vi "WheelShooter Load Data.vi"(1 "error in":errorcluster, 2 "Range":dbl) -> (0 "cluster":T9)   [LabVIEW 2015]
uses:
  <vilib>/Rock Robotics/WPI/MotorControl/WPI_MotorControlDeviceRef.ctl
  <vilib>/Rock Robotics/WPI/MotorControl/WPI_MotorControlType.ctl
  <vilib>/Rock Robotics/SystemInterfaces/DIO/FPGA_DIOPWMChannel.ctl
  <vilib>/Rock Robotics/WPI/PWM/WPI_PWMDeadband.ctl
  <vilib>/Rock Robotics/WPI/CAN/Jaguar/SubVIs/WPI_CANJaguar_ControlMode.ctl
  <vilib>/Rock Robotics/WPI/CAN/TalonSRX/WPI_CANTalonSRX_APIControlMode.ctl
  <vilib>/Rock Robotics/WPI/PWM/Servo/WPI_ServoDeviceRef.ctl
  <vilib>/Utility/file.llb/Read Delimited Spreadsheet (DBL).vi
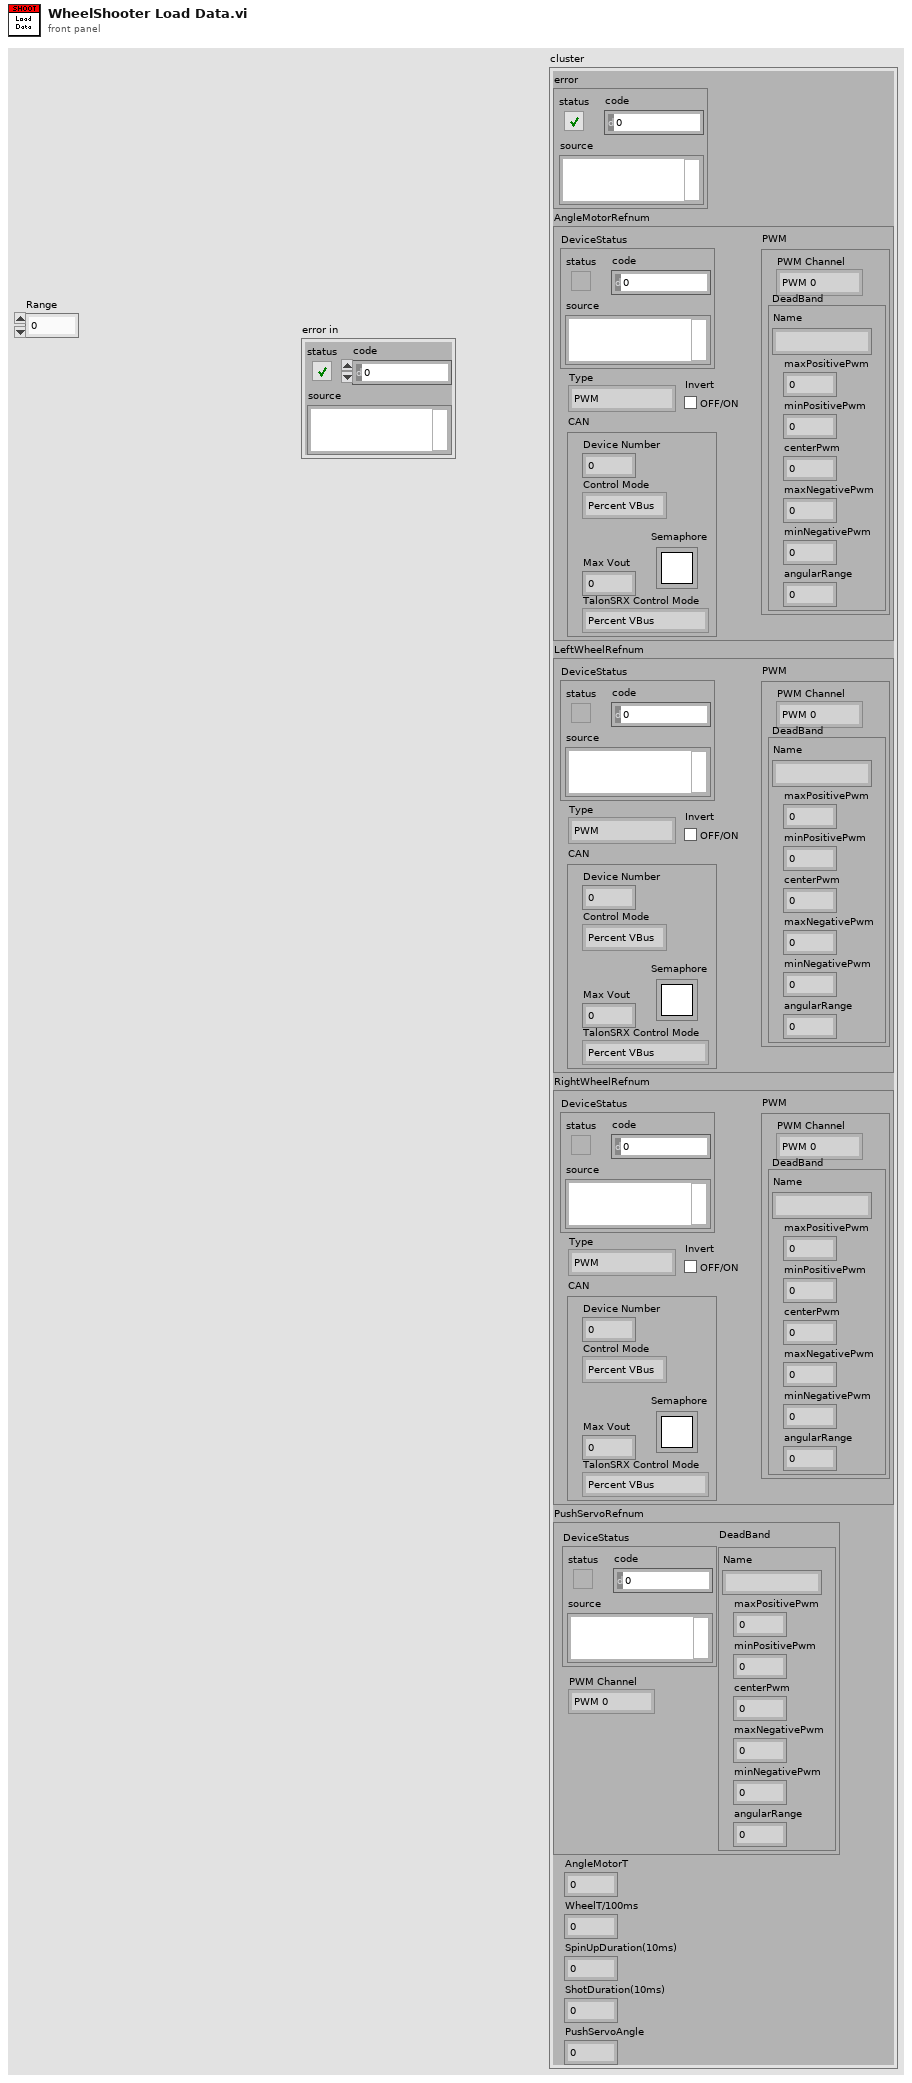
[diagram p1: front panel]
types:
  T1 = typedef "WPI_MotorControlDeviceRef.ctl" = cluster{"DeviceStatus":errorcluster, "Type":T2, "PWM":cluster{"PWM Channel":T3, "DeadBand":T4}, "CAN":cluster{"Device Number":u8, "Control Mode":T5, "Semaphore":T6, "Max Vout":dbl, "TalonSRX Control Mode":T7}, "Invert":bool}
  T2 = typedef "WPI_MotorControlType.ctl" = enum16{"PWM", "CAN", "CANTalonSRX"}
  T3 = typedef "FPGA_DIOPWMChannel.ctl" = enum8{"PWM 0", "PWM 1", "PWM 2", "PWM 3", "PWM 4", "PWM 5", "PWM 6", "PWM 7", "PWM 8", "PWM 9", "PWM MXP 0", "PWM MXP 1", "PWM MXP 2", "PWM MXP 3", "PWM MXP 4", "PWM MXP 5", "PWM MXP 6", "PWM MXP 7", "PWM MXP 8", "PWM MXP 9", "Invalid"}
  T4 = typedef "WPI_PWMDeadband.ctl" = cluster{"Name":string, "maxPositivePwm":i32, "minPositivePwm":i32, "centerPwm":i32, "maxNegativePwm":i32, "minNegativePwm":i32, "angularRange":u16}
  T5 = typedef "WPI_CANJaguar_ControlMode.ctl" = enum8{"Percent VBus", "Current", "Speed", "Position", "Voltage"}
  T6 = typedef "Semaphore RefNum" = refnum<k1>
  T7 = typedef "WPI_CANTalonSRX_APIControlMode.ctl" = enum8{"Percent VBus", "Speed", "Position", "Slave", "Unchanged / Invalid", "Voltage Compensation", "Current", "Motion Profile"}
  T8 = typedef "WPI_ServoDeviceRef.ctl" = cluster{"DeviceStatus":errorcluster, "PWM Channel":T3, "DeadBand":T4}
  T9 = cluster{"error":errorcluster, "AngleMotorRefnum":T1, "LeftWheelRefnum":T1, "RightWheelRefnum":T1, "PushServoRefnum":T8, "AngleMotorT":dbl, "WheelT/100ms":dbl, "SpinUpDuration(10ms)":i32, "ShotDuration(10ms)":i32, "PushServoAngle":i32}
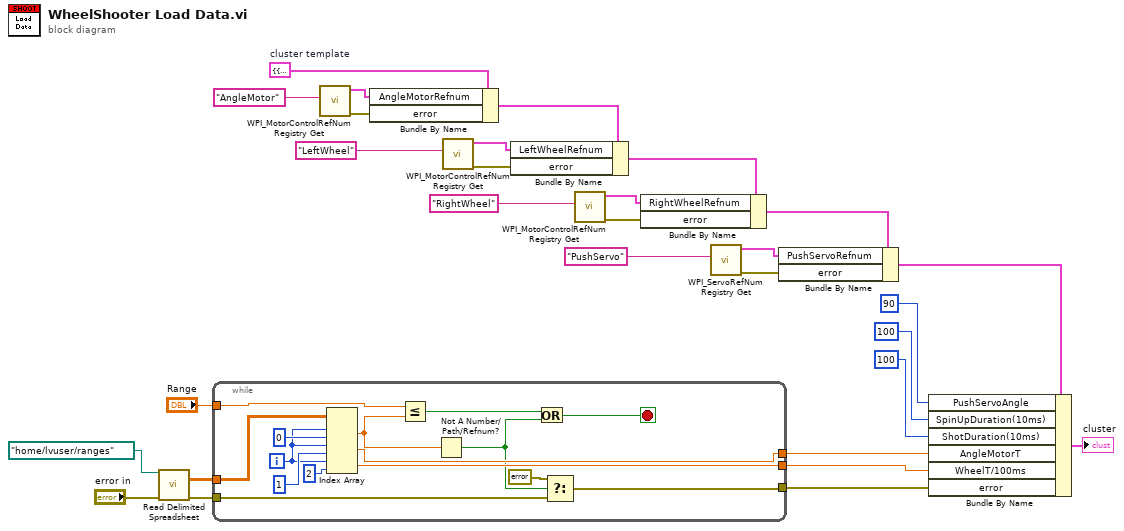
[diagram p0: block diagram]
diagram:
  w3 = T9 {"error"={"status"=FALSE, "code"=0, "source"=""}, "AngleMotorRefnum"={"DeviceStatus"={"status"=FALSE, "code"=0, "source"=""}, "Type"=enum."PWM", "PWM"={"PWM Channel"=enum."Invalid", "DeadBand"={"Name"="", "maxPositivePwm"=0, "minPositivePwm"=0, "centerPwm"=0, "maxNegativePwm"=0, "minNegativePwm"=0, "angularRange"=0}}, "CAN"={"Device Number"=0, "Control Mode"=enum."Percent VBus", "Semaphore"=refnum, "Max Vout"=12.0, "TalonSRX Control Mode"=enum."Percent VBus"}, "Invert"=FALSE}, "LeftWheelRefnum"={"DeviceStatus"={"status"=FALSE, "code"=0, "source"=""}, "Type"=enum."PWM", "PWM"={"PWM Channel"=enum."Invalid", "DeadBand"={"Name"="", "maxPositivePwm"=0, "minPositivePwm"=0, "centerPwm"=0, "maxNegativePwm"=0, "minNegativePwm"=0, "angularRange"=0}}, "CAN"={"Device Number"=0, "Control Mode"=enum."Percent VBus", "Semaphore"=refnum, "Max Vout"=12.0, "TalonSRX Control Mode"=enum."Percent VBus"}, "Invert"=FALSE}, "RightWheelRefnum"={"DeviceStatus"={"status"=FALSE, "code"=0, "source"=""}, "Type"=enum."PWM", "PWM"={"PWM Channel"=enum."Invalid", "DeadBand"={"Name"="", "maxPositivePwm"=0, "minPositivePwm"=0, "centerPwm"=0, "maxNegativePwm"=0, "minNegativePwm"=0, "angularRange"=0}}, "CAN"={"Device Number"=0, "Control Mode"=enum."Percent VBus", "Semaphore"=refnum, "Max Vout"=12.0, "TalonSRX Control Mode"=enum."Percent VBus"}, "Invert"=FALSE}, "PushServoRefnum"={"DeviceStatus"={"status"=FALSE, "code"=0, "source"=""}, "PWM Channel"=enum."Invalid", "DeadBand"={"Name"="", "maxPositivePwm"=0, "minPositivePwm"=0, "centerPwm"=0, "maxNegativePwm"=0, "minNegativePwm"=0, "angularRange"=0}}, "AngleMotorT"=0.0, "WheelT/100ms"=0.0, "SpinUpDuration(10ms)"=0, "ShotDuration(10ms)"=0, "PushServoAngle"=0}  # cluster template
  n1 = call-poly <vilib>:"Read Delimited Spreadsheet.vi"("file path (dialog if empty)"=path "/home/lvuser/ranges", "error in (no error)"="error in") -> ("all rows"=w28:dbl[][], "error out"=w27:errorcluster)  [unwired: 8 in, 4 out]
  n2 = while {
    tunnel: "Range" -> [w37]
    tunnel: [w41] -> w9
    tunnel: [w40] -> w10
    tunnel: w28 -> [w39]
    tunnel: w27 -> [w30]
    tunnel: [w31] -> w11
    i -> [w38]
    stop <- w34 stop-if-true
    n3 = Index Array(array=w39, index (row) #1=w38, index (col) #1=0 ("disabled index (col)"), index (row) #2=w38, index (col) #2=1 ("disabled index (col)"), index (row) #3=w38, index (col) #3=2 ("disabled index (col)")) -> (element #1=w36:dbl, element #2=w41:dbl, element #3=w40:dbl)
    n4 = Less Or Equal?(x=w37, y=w36) -> (x <= y?=w35:bool)
    n5 = Not A Number/Path/Refnum?(number/path/refnum=w36) -> (NaN/Path/Refnum?=w32:bool)
    n6 = Or(x=w35, y=w32) -> (x .or. y?=w34:bool)
    n7 = Select(t=errorcluster {"status"=TRUE, "code"=9001, "source"="Out of range!"} ("error constant"), s=w32, f=w30) -> (s? t:f=w31:errorcluster)
  }
  n8 = call <vilib>:"WPI_MotorControlRefNum Registry Get.vi"("refnum name"="AngleMotor") -> ("error out"=w18:errorcluster, "MotorControlDevRef"=w22:T1)  [unwired: 9 in]
  n9 = Bundle By Name(cluster=w3, "AngleMotorRefnum"=w22, "error"=w18) -> (w15:T9)
  n10 = call <vilib>:"WPI_MotorControlRefNum Registry Get.vi"("refnum name"="LeftWheel") -> ("error out"=w16:errorcluster, "MotorControlDevRef"=w20:T1)  [unwired: 9 in]
  n11 = Bundle By Name(cluster=w15, "LeftWheelRefnum"=w20, "error"=w16) -> (w14:T9)
  n12 = call <vilib>:"WPI_MotorControlRefNum Registry Get.vi"("refnum name"="RightWheel") -> ("error out"=w17:errorcluster, "MotorControlDevRef"=w21:T1)  [unwired: 9 in]
  n13 = Bundle By Name(cluster=w14, "RightWheelRefnum"=w21, "error"=w17) -> (w13:T9)
  n14 = call <vilib>:"WPI_ServoRefNum Registry Get.vi"("refnum name"="PushServo") -> ("error out"=w12:errorcluster, "ServoDeviceRef"=w19:T8)  [unwired: 9 in]
  n15 = Bundle By Name(cluster=w13, "PushServoRefnum"=w19, "error"=w12) -> (w8:T9)
  n16 = Bundle By Name(cluster=w8, "PushServoAngle"=90, "SpinUpDuration(10ms)"=100, "ShotDuration(10ms)"=100, "AngleMotorT"=w9, "WheelT/100ms"=w10, "error"=w11) -> (→"cluster":T9)
